vi "stop.vi"(8 "error in (no error)":errorcluster, 11 "librarian_sm in":refnum<class "client.lvclass">) -> (0 "error out":errorcluster, 3 "librarian_sm out":refnum<class "client.lvclass">)   [LabVIEW 2020, in "client.lvclass"]
uses:
  client.lvclass
  client.lvclass/client.ctl
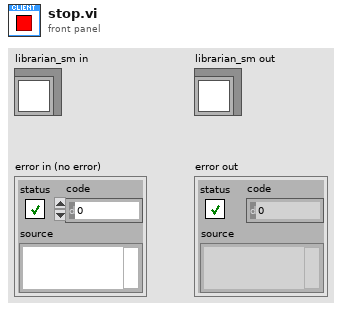
[diagram p1: front panel]
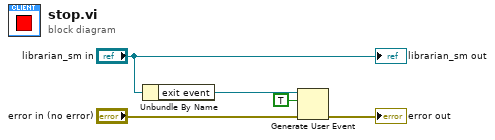
[diagram p0: block diagram]
diagram:
  n1 = Unbundle By Name("librarian_sm in") -> ("exit event"=w5:refnum<user-event>)
  n2 = Generate User Event(user event=w5, event data cluster=TRUE ("event data"), error in="error in (no error)") -> (error out=→"error out":errorcluster)  [unwired: 1 in, 1 out]
  "librarian_sm out" <- "librarian_sm in"
